vi "dfd_DFXP_DFXP to Double (vector).vi"(10 "Value in":T1) -> (2 "DBL":dbl[](array[numeric]))   [LabVIEW 2017, in "NI_DigFilter_FXP.lvlib"]
uses:
  <vilib>/addons/Digital Filter Design/NI_DigFilter_FXP.lvlib
  <vilib>/addons/Digital Filter Design/_Objects.llb/dfd_DFXP Data Type (vector).ctl
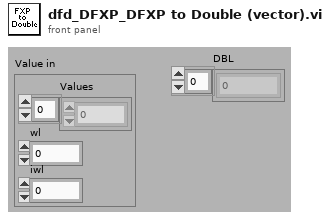
[diagram p1: front panel]
types:
  T1 = typedef "dfd_DFXP Data Type (vector).ctl" = cluster{"Values":i64[], "wl":i16, "iwl":i16}
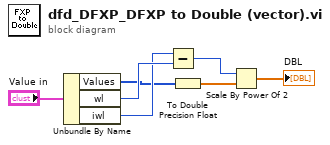
[diagram p0: block diagram]
diagram:
  n1 = Unbundle By Name("Value in") -> ("Values"=w3:i64[], "wl"=w5:i16, "iwl"=w4:i16)
  n2 = Subtract(x=w4, y=w5) -> (x-y=w6:i16)
  n3 = To Double Precision Float(number=w3) -> (double precision float=w7:dbl[])
  n4 = Scale By Power Of 2(n=w6, x=w7) -> (x*2^n=→"DBL":dbl[])
